vi "ICM Find Serial Ports.vi"() -> (3 "Serial Ports":i32[](array[numeric]))   [LabVIEW 2018]
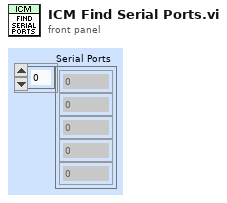
[diagram p1: front panel]
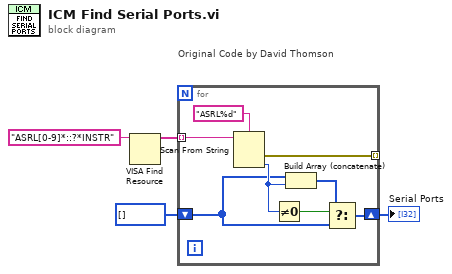
[diagram p0: block diagram]
diagram:
  n1 = VISA Find Resource(11:"ASRL[0-9]*::?*INSTR" ("expression (\"?*\")")) -> (3:w2:string[])  [unwired: 2 in, 2 out]
  n2 = for "Original Code by David Thomson" {
    tunnel: w2 -> [w12] mode=indexing
    tunnel: [w11] -> _ mode=indexing
    shift-right: [w8] -> w4
    shift-left: i32[] [] -> [w6]
    n3 = Scan From String(format string="ASRL%d", input string=w12) -> (error out=w11:errorcluster, output 1=w7:i32)  [unwired: 3 in, 2 out]
    n4 = Not Equal To 0?(x=w7) -> (x != 0?=w9:bool)
    n5 = Build Array (concatenate)(w6, w7) -> (w5:i32[])
    n6 = Select(t=w5, s=w9, f=w6) -> (s? t:f=w8:i32[])
  }
  "Serial Ports" <- w4
